vi "_CheckPasswordLegal.vi"(8 "error in (no error)":errorcluster, 11 "Password":string) -> (0 "error out":errorcluster, 2 "legal?":bool)   [LabVIEW 2017, in "Login-UI.lvlib"]
uses:
  Login-UI.lvlib
  <vilib>/regexp/Match Regular Expression.xnode
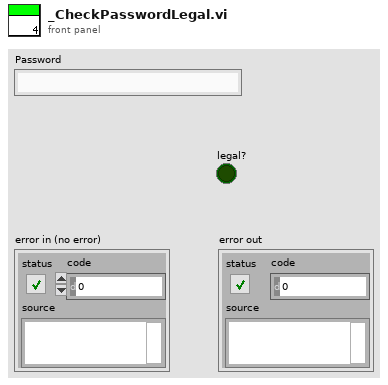
[diagram p1: front panel]
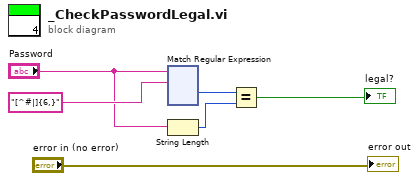
[diagram p0: block diagram]
diagram:
  n1 = xnode "Match Regular Expression"("input string"="Password", "regular expression"="[^#|]{6,}") -> ("offset past match"=w4:i32)  [unwired: 4 in, 4 out]
  n2 = String Length(string="Password") -> (length=w2:i32)
  n3 = Equal?(x=w4, y=w2) -> (x = y?=→"legal?":bool)
  "error out" <- "error in (no error)"
